vi "Address Test.vi"() -> ()   [LabVIEW 2013]
uses:
  <vilib>/rvi/DataTransferAndStorage/Container/XNode/niFpgaContainer.xnode
  <vilib>/rvi/Memory/Memory_Emulation/nirvimemoryFastEmulation.vi
  <vilib>/rvi/Memory/Memory_Emulation/nirvimemoryEmulation.vi
panel:
  out "Buffer Addresses Read":i32[](graph)
  out "Data in Buffer":i32[](graph)
  in  "Value to Stop Test":i32
  # "Overview: This example demonstrates the logic for using block memory to act as a circular buffer for FPGA.\nRequirenments: LabVIEW 2013 or compatible\nInstructions:\n1. Open the Test Buffer LabVIEW Project and the Address Test VI.\n2. Enter a desired value into the numeric control (anything between 0 and 20,000 will return valid results).\n3. Run the VI to simulate the FPGA operation and populate the graphs."
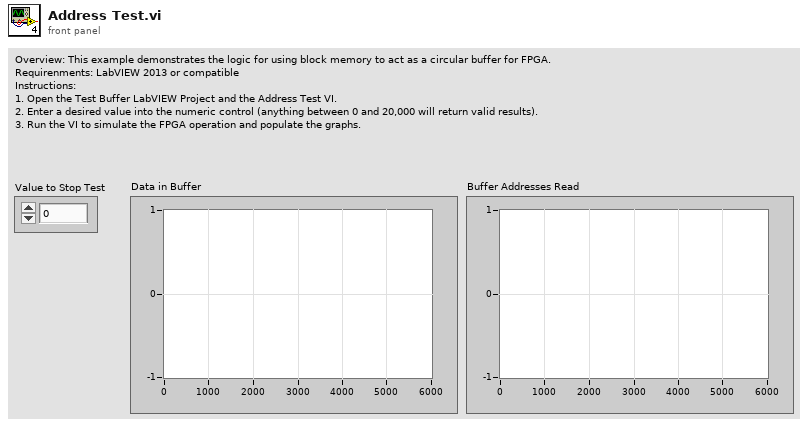
[diagram p1: front panel]
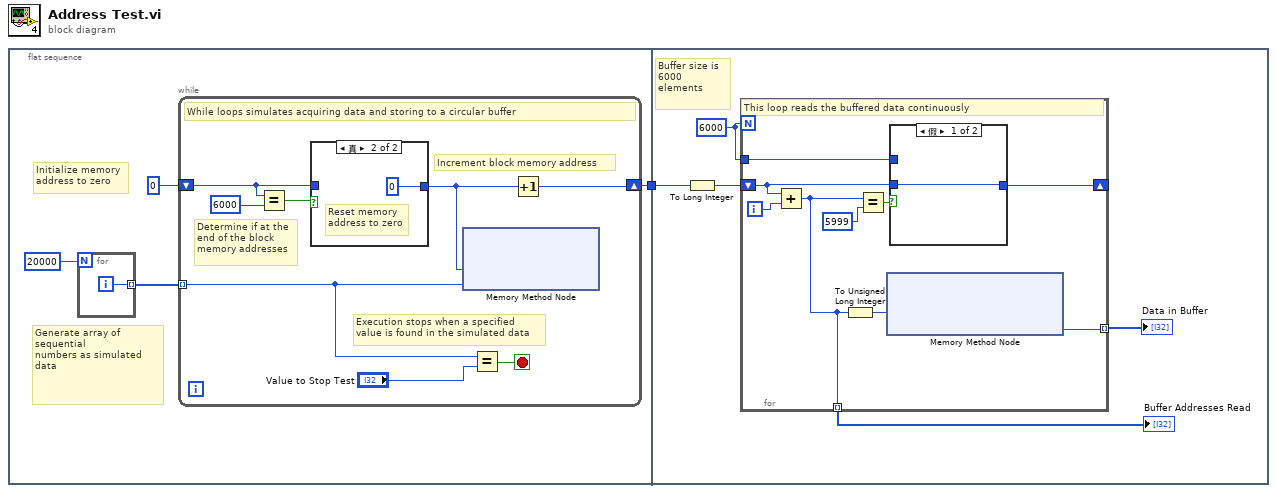
[diagram p0: block diagram]
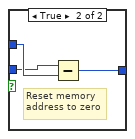
[diagram p3: hidden frame]
diagram:
  n1 = flat-sequence {
    tunnel: [w2] -> w1
    tunnel: w1 -> [w21]
    frame #0 {
      # "Initialize memory\naddress to zero"
      # "Generate array of sequential\nnumbers as simulated data"
      n2 = for {
        N: 20000 -> [_]
        tunnel: [w6] -> w3 mode=indexing
        i -> [w6]
      }
      n3 = while {
        shift-right: [w14] -> w2
        shift-left: u32 0 -> [w11]
        tunnel: w3 -> [w9] mode=indexing
        stop <- w8 stop-if-true
        # "Increment block memory address"
        # "Determine if at the\nend of the block\nmemory addresses"
        # "Execution stops when a specified\nvalue is found in the simulated data"
        # "While loops simulates acquiring data and storing to a circular buffer"
        n4 = Equal?(x=w11, y=u32 6000) -> (x = y?=w12:bool)
        n5 = case shown="真" w12 {
          tunnel: w11 -> [w15 _]
          tunnel: [w15 u32 0] -> w10
          frame False {
          }
          frame True {
            # "Reset memory\naddress to zero"
          }
        }
        n6 = xnode "Memory Method Node"("地址"=w10, "数据"=w9) -> ()  [unwired: 1 in, 1 out]
        n7 = Equal?(x=w9, y="Value to Stop Test") -> (x = y?=w8:bool)
        n8 = Increment(x=w10) -> (x+1=w14:u32)
      }
    }
    frame #1 {
      w19 = 6000
      # "Buffer size is 6000 elements"
      n9 = To Long Integer(number=w21) -> (32bit integer=w20:i32)
      n10 = for {
        N: w19 -> [_]
        tunnel: [w30] -> w18 mode=indexing
        shift-right: [w27] -> _
        shift-left: w20 -> [w28]
        tunnel: w19 -> [w24]
        tunnel: [w22] -> w17 mode=indexing
        i -> [w26]
        # "This loop reads the buffered data continuously"
        n11 = Add(x=w28, y=w26) -> (x+y=w22:i32)
        n12 = To Unsigned Long Integer(number=w22) -> (unsigned 32bit integer=w25:u32)
        n13 = Equal?(x=w22, y=u32 5999) -> (x = y?=w29:bool)
        n14 = xnode "Memory Method Node"("地址"=w25) -> ("数据"=w30:i32)  [unwired: 1 in, 1 out]
        n15 = case shown="假" w29 {
          tunnel: w28 -> [w31 w32]
          tunnel: [w31 w33] -> w27
          tunnel: w24 -> [_ w34]
          frame False {
          }
          frame True {
            # "Reset memory\naddress to zero"
            n16 = Subtract(x=w32, y=w34) -> (x-y=w33:i32)
          }
        }
      }
      "Data in Buffer" <- w18
      "Buffer Addresses Read" <- w17
    }
  }
